vi "Set System Explorer Busy.vi"(8 "error in (no error)":errorcluster) -> (0 "error out":errorcluster)   [LabVIEW 2020, in "SLSC EDS System Explorer.lvlib"]
uses:
  SLSC EDS System Explorer.lvlib
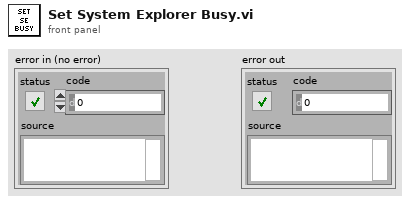
[diagram p1: front panel]
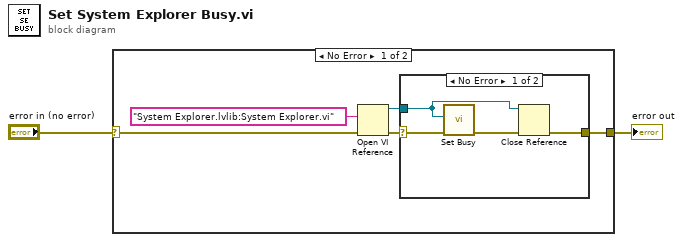
[diagram p0: block diagram]
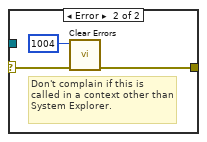
[diagram p2: hidden frame]
diagram:
  n1 = case shown="No Error" "error in (no error)" {
    selector: "error in (no error)" -> [w3 w15]
    tunnel: [w4 w15] -> w2
    frame No Error {
      n2 = Open VI Reference(vi path="System Explorer.lvlib:System Explorer.vi", error in (no error)=w3) -> (vi reference=w5:refnum<vi>, error out=w6:errorcluster)  [unwired: 4 in]
      n3 = case shown="No Error" w6 {
        selector: w6 -> [w11 w14]
        tunnel: w5 -> [w9 _]
        tunnel: [w8 w13] -> w4
        frame No Error {
          n4 = call <vilib>:"Set Busy.vi"("error in (no error)"=w11, "VI reference (current VI)"=w9) -> ("error out"=w10:errorcluster)  [unwired: 8 in, 1 out]
          n5 = Close Reference(reference=w9, error in (no error)=w10) -> (error out=w8:errorcluster)
        }
        frame Error {
          # "Don't complain if this is called in a context other than System Explorer."
          n6 = call <vilib>:"Clear Errors.vi"("error in (no error)"=w14, "specific error code to clear (0: all)"=1004) -> ("error out"=w13:errorcluster)  [unwired: 4 in, 1 out]
        }
      }
    }
    frame Error {
    }
  }
  "error out" <- w2
